vi "Move.vi"(8 "error in":errorcluster, 9 "Y":i32, 10 "X":i32, 11 "Uno in":refnum<class "Uno.lvclass">) -> (0 "error out":errorcluster, 3 "Uno out":refnum<class "Uno.lvclass">)   [LabVIEW 2020, in "Uno.lvclass"]
uses:
  Uno.lvclass
  Uno.lvclass/Uno.ctl
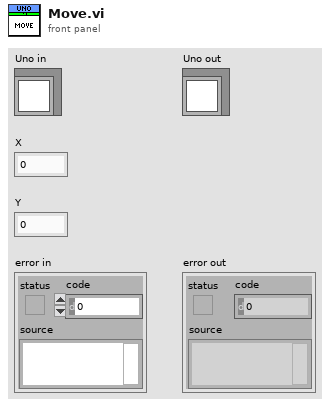
[diagram p1: front panel]
types:
  T1 = typedef "Uno.lvclass/Group Data.ctl" = cluster{"our positions":u8[][]}
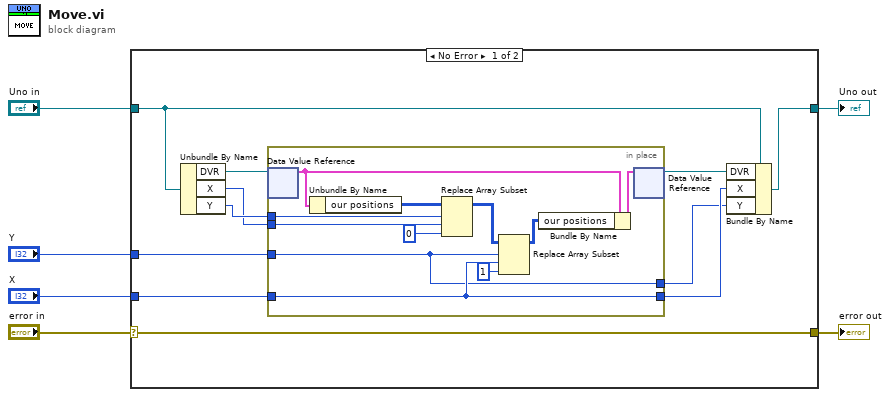
[diagram p0: block diagram]
diagram:
  n1 = case shown="No Error" "error in" {
    selector: "error in" -> [w17 w30]
    tunnel: [w17 w30] -> w5
    tunnel: [w15 w29] -> w3
    tunnel: "Uno in" -> [w16 w29]
    tunnel: "Y" -> [w12 _]
    tunnel: "X" -> [w11 _]
    frame No Error {
      n2 = Unbundle By Name(w16) -> ("DVR"=w13:refnum<data-value>, "X"=w9:i32, "Y"=w10:i32)
      n3 = in-place {
        in-place-border: w12 -> [w20]
        in-place-border: w11 -> [w21]
        in-place-border: w10 -> [w23]
        in-place-border: w9 -> [w22]
        in-place-border: [w21] -> w8
        in-place-border: [w20] -> w7
        n4 = in-place-dvr #1(w13) -> (w28:T1)  [unwired: 1 out]
        n5 = Unbundle By Name(w28) -> ("our positions"=w25:u8[][])
        n6 = Replace Array Subset(array=w25, new element=u8 0 ("new element/subarray"), index (row)=w23, index (col)=w22) -> (w24:u8[][])
        n7 = Replace Array Subset(array=w24, new element=u8 1 ("new element/subarray"), index (row)=w20, index (col)=w21) -> (w26:u8[][])
        n8 = Bundle By Name(cluster=w28, "our positions"=w26) -> (w27:T1)
        n9 = in-place-dvr #1(w27) -> (w14:refnum<data-value>)  [unwired: 1 out]
      }
      n10 = Bundle By Name(cluster=w16, "DVR"=w14, "X"=w8, "Y"=w7) -> (w15:refnum<class "Uno.lvclass">)
    }
    frame Error {
    }
  }
  "error out" <- w5
  "Uno out" <- w3
